vi "Day07-2.vi"() -> ()   [LabVIEW 2021]
uses:
  f00bd700-c5e9-4b99-81d8-9b982d1785ce.vi
panel:
  out "Total Fuel Needed":i64
  out "input values":i64[](array[numeric])
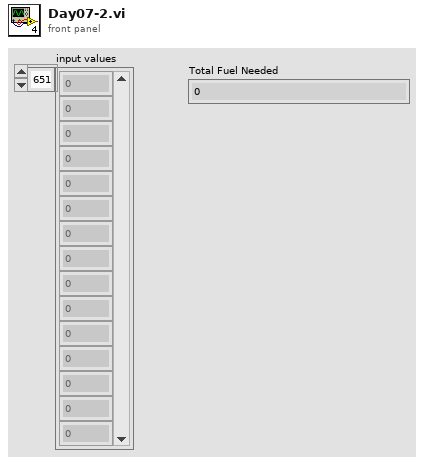
[diagram p1: front panel]
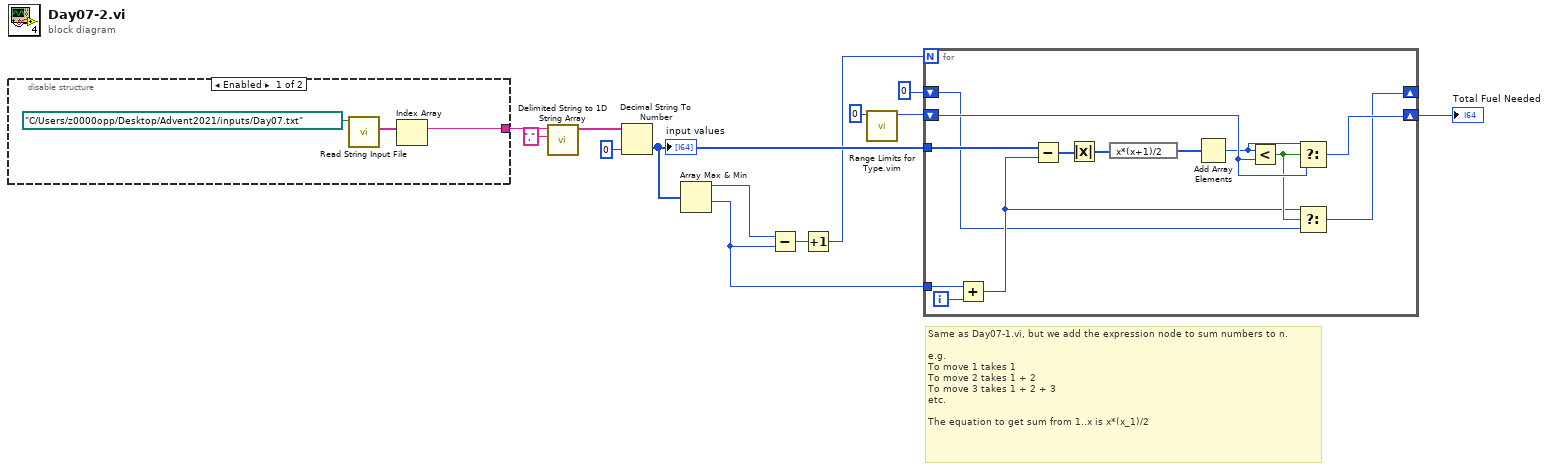
[diagram p0: block diagram]
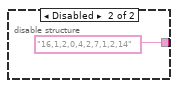
[diagram p2: hidden frame]
diagram:
  # "Same as Day07-1.vi, but we add the expression node to sum numbers to n.\n\ne.g.\nTo move 1 takes 1\nTo move 2 takes 1 + 2\nTo move 3 takes 1 + 2 + 3\netc.\n\nThe equation to get sum from 1..x is x*(x_1)/2"
  n1 = disable-structure shown="Enabled" {
    disable-tunnel: [w14 "16,1,2,0,4,2,7,1,2,14" ("String")] -> w10
    frame Enabled {
      n2 = call "Read String Input File.vi"("file path (dialog if empty)"=path "C:/Users/z0000opp/Desktop/Advent2021/inputs/Day07.txt") -> ("input values"=w15:string[])  [unwired: 10 in]
      n3 = Index Array(array=w15) -> (element=w14:string)  [unwired: 1 in]
    }
    frame Disabled {
    }
  }
  n4 = call <vilib>:"Delimited String to 1D String Array.vi"("delimiter"=",", "delimited string"=w10) -> ("string array"=w13:string[])  [unwired: 9 in]
  n5 = Decimal String To Number(string=w13, default (0L)=i64 0 ("default (0 I32)")) -> (number=w9:i64[])  [unwired: 1 in, 1 out]
  "input values" <- w9
  n6 = Array Max & Min(array=w9) -> (max value=w8:i64, min value=w5:i64)  [unwired: 2 out]
  n7 = Subtract(x=w8, y=w5) -> (x-y=w7:i64)
  n8 = Increment(x=w7) -> (x+1=w6:i64)
  n9 = call "Range Limits for Type.vim"("type"=0) -> ("maximum value for type"=w3:i32)  [unwired: 9 in, 1 out]
  n10 = for {
    N: w6 -> [_]
    tunnel: w9 -> [w28]
    tunnel: w5 -> [w29]
    shift-right: [w21] -> _
    shift-left: 0 -> [w20]
    shift-right: [w24] -> w1
    shift-left: w3 -> [w26]
    i -> [w30]
    n11 = Add(x=w29, y=w30) -> (x+y=w22:i64)
    n12 = Subtract(x=w28, y=w22) -> (x-y=w27:i64[])
    n13 = Absolute Value(x=w27) -> (abs(x)=w19:i64[])
    n14 = expression code="x*(x+1)/2"(w19) -> (w18:i64[])
    n15 = Add Array Elements(numeric array=w18) -> (sum=w25:i64)
    n16 = Less?(x=w25, y=w26) -> (x < y?=w23:bool)
    n17 = Select(t=w25, s=w23, f=w26) -> (s? t:f=w24:i64)
    n18 = Select(t=w22, s=w23, f=w20) -> (s? t:f=w21:i64)
  }
  "Total Fuel Needed" <- w1
